vi "CIC_downsample_configurable.vi"(7 "new rate":fxp<+,8,8>, 8 "valid in":bool, 10 "din":fxp<+/-,20,16>, 11 "rate change":bool) -> (0 "valid out":bool, 1 "rdy for data":bool, 2 "dout":fxp<+/-,25,19>)   [LabVIEW 2013]
uses:
  <vilib>/rvi/FXPMathLib/FxpConvert/subVIs/nifxpmath_Convert_SimConfig.ctl
  <vilib>/fxp/LVFixedPointQuantizationPolicyTypeDef.ctl
  <vilib>/fxp/LVFixedPointOverflowPolicyTypeDef.ctl
  <vilib>/rvi/FXPMathLib/FxpConvert/simVIs/DllFxpConvertTemp_sub.vi
  <vilib>/rvi/IPIntegrationNode/IPINode_Utilities/niFpgaIPINodeSimCore.vi
  <vilib>/rvi/FXPMathLib/FxpConvert/XNode/nifxpmath_Convert.xnode
  <vilib>/rvi/XilinxIP/XIPIN_XNode/niFpgaXIPIN.xnode
  Xilinx compiled/CIC_reconfig/CIC_Reconfig_BD6D03573A4E4F6FB3406D1CDE9F6D91.dll
  <vilib>/rvi/IPIntegrationNode/IPINode_Xnode/niFpgaIPINode.xnode
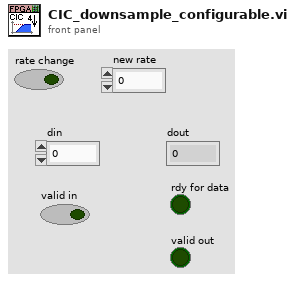
[diagram p1: front panel]
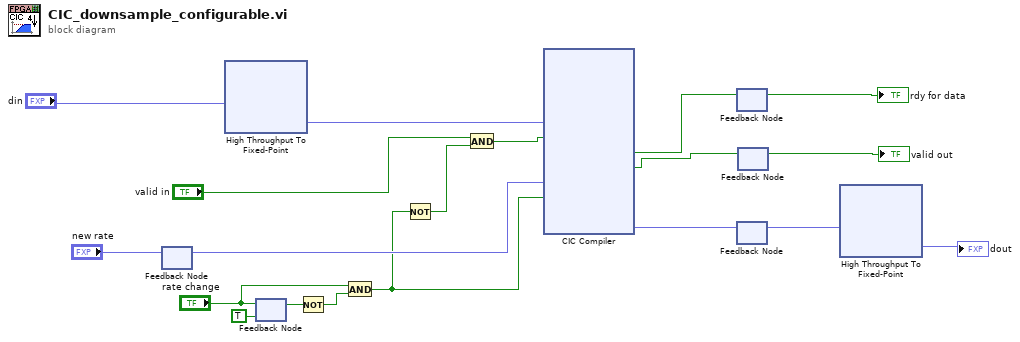
[diagram p0: block diagram]
diagram:
  n1 = feedback #1() -> (w6:fxp<+,8,8>)  [unwired: 1 in]
  n2 = feedback-in #1("new rate") -> ()
  n3 = xnode "High Throughput To Fixed-Point"("x"="din") -> ("y"=w11:fxp<+/-,24,20>)
  n4 = feedback-in #2("rate change") -> ()
  n5 = feedback #2(TRUE ("rate change")) -> (w16:bool)
  n6 = Not(x=w16) -> (.not. x?=w14:bool)
  n7 = And(x="rate change", y=w14) -> (x .and. y?=w4:bool)
  n8 = Not(x=w4) -> (.not. x?=w5:bool)
  n9 = And(x="valid in", y=w5) -> (x .and. y?=w3:bool)
  n10 = xnode ("CIC Compiler")("s_axis_data_tdata"=w11, "s_axis_data_tvalid"=w3, "s_axis_config_tdata"=w6, "s_axis_config_tvalid"=w4) -> ("s_axis_data_tready"=w10:bool, "m_axis_data_tvalid"=w9:bool, "m_axis_data_tdata"=w8:fxp<+/-,40,26>)  [unwired: 2 in, 1 out]
  n11 = feedback #3() -> (→"rdy for data":bool)  [unwired: 1 in]
  n12 = feedback-in #3(w10) -> ()
  n13 = feedback #4() -> (w2:fxp<+/-,40,26>)  [unwired: 1 in]
  n14 = feedback-in #4(w8) -> ()
  n15 = feedback #5() -> (→"valid out":bool)  [unwired: 1 in]
  n16 = feedback-in #5(w9) -> ()
  n17 = xnode "High Throughput To Fixed-Point"("x"=w2) -> ("y"=→"dout":fxp<+/-,25,19>)
